vi "CLI_Write Nipkg Metadata.vi"(11 "CLI Arguments":string[](array[string])) -> (2 "Output":string, 3 "Error Code":i32)   [LabVIEW 2014]
doc: "Copyright (c) 2018 Sze Howe Koh\n\nThis Source Code Form is subject to the terms of the Mozilla Public License, v. 2.0. If a copy of the MPL was not distributed with this file, You can obtain one at http://mozilla.org/MPL/2.0/."
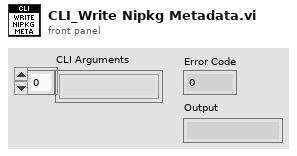
[diagram p1: front panel]
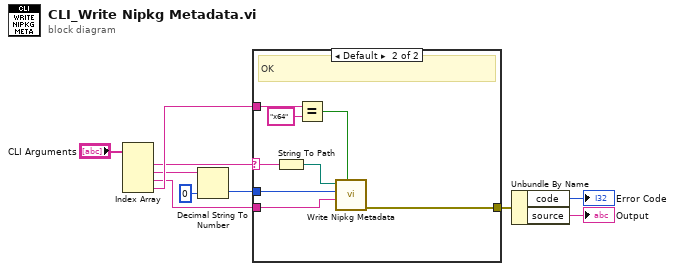
[diagram p0: block diagram]
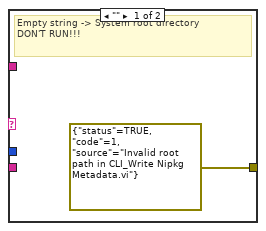
[diagram p2: hidden frame]
diagram:
  n1 = Index Array(array="CLI Arguments") -> (element #1=w8:string, element #2=w4:string, element #3=w2:string, element #4=w10:string)  [unwired: 4 in]
  n2 = Decimal String To Number(string=w4, default (0L)=u16 0 ("default (0 I32)")) -> (number=w3:u16)  [unwired: 1 in, 1 out]
  n3 = case shown="Default" w8 {
    selector: w8 -> [_ w19]
    tunnel: [errorcluster {"status"=TRUE, "code"=1, "source"="Invalid root path in CLI_Write Nipkg Metadata.vi"} w17] -> w7
    tunnel: w10 -> [_ w16]
    tunnel: w3 -> [_ w13]
    tunnel: w2 -> [_ w12]
    frame "" {
      # "Empty string -> System root directory\nDON'T RUN!!!"
    }
    frame Default {
      # "OK"
      n4 = String To Path(string=w19) -> (path=w18:path)
      n5 = Equal?(x=w16, y="x64") -> (x = y?=w14:bool)
      n6 = call "Write Nipkg Metadata.vi"("64-bit?"=w14, "Package Version"=w12, "LabVIEW Version"=w13, "Root Folder"=w18) -> ("Error Out"=w17:errorcluster)  [unwired: 7 in]
    }
  }
  n7 = Unbundle By Name(w7) -> ("code"=→"Error Code":i32, "source"=→"Output":string)
